vi "Send Write Setup.vi"(8 "error in (no error)":errorcluster, 11 "RxTx in":refnum<class "RxTx.lvclass">) -> (0 "error out":errorcluster, 3 "RxTx out":refnum<class "RxTx.lvclass">)   [LabVIEW 2018, in "RxTx.lvclass"]
uses:
  RxTx.lvclass
  RxTx.lvclass/RxTx.ctl
  Interface/Interface.lvclass
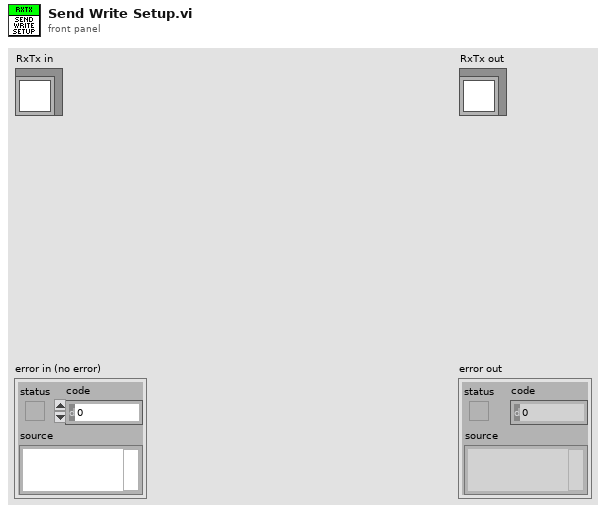
[diagram p1: front panel]
types:
  T1 = cluster{"Exposure Time":sgl, "Pre-amp gain":u8, "Readout Rate":u8, "EM Mode":u8, "EM Gain":u16, "Binning":u16, "Initial Line":u16, "Initial Cloumn":u16, "Final Line":u16, "Final Column":u16, "Kinetic Series Length":u32, "Shutter Mode":u8, "Cooler ON/OFF":u16, "Temperature":i8, "Cubes":u32, "Trigger":u16}
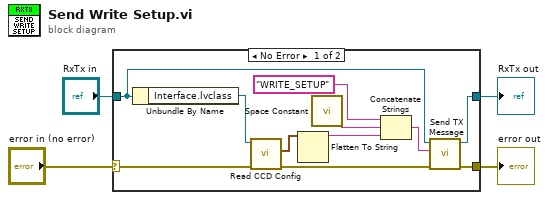
[diagram p0: block diagram]
diagram:
  n1 = case shown="No Error" "error in (no error)" {
    selector: "error in (no error)" -> [w14 w17]
    tunnel: [w8 w17] -> w2
    tunnel: [w9 w16] -> w1
    tunnel: "RxTx in" -> [w10 w16]
    frame No Error {
      n2 = Unbundle By Name(w10) -> ("Interface.lvclass"=w15:refnum<class "Interface.lvclass">)
      n3 = call "Read CCD Config.vi"("error in (no error)"=w14, "Interface in"=w15) -> ("error out"=w12:errorcluster, "CCD Config"=w6:T1)  [unwired: 7 in, 1 out]
      n4 = Flatten To String(anything=w6) -> (data string=w13:string)  [unwired: 3 in, 2 out]
      n5 = call <vilib>:"Space Constant.vi"() -> ("String"=w7:string)
      n6 = Concatenate Strings("WRITE_SETUP", w7, w13) -> (w11:string)
      n7 = call "Send TX Message.vi"("error in (no error)"=w12, "element"=w11, "RxTx in"=w10) -> ("error out"=w8:errorcluster, "RxTx out"=w9:refnum<class "RxTx.lvclass">)  [unwired: 7 in]
    }
    frame Error {
    }
  }
  "error out" <- w2
  "RxTx out" <- w1
